vi "GEA2 Log Filter.vi"(0 "Filter Log":bool, 5 "Filter Data":bool, 7 "GEA2 Msg":T1 {"Command" format="%02x"; "Destination" format="%02x"; "Source" format="%02x"}, 9 "Cmd to Filter":string, 11 "error in (no error)":errorcluster) -> (15 "error out":errorcluster)   [LabVIEW 2021]
uses:
  Common/LabVIEW GEA2 Toolkit/GEA3/type defs/Data In.ctl
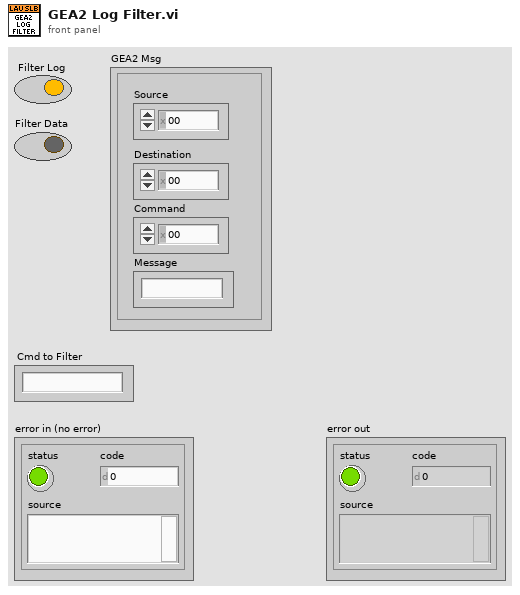
[diagram p1: front panel]
types:
  T1 = typedef "Data In.ctl" = cluster{"Source":u8, "Destination":u8, "Command":u8, "Message":string}
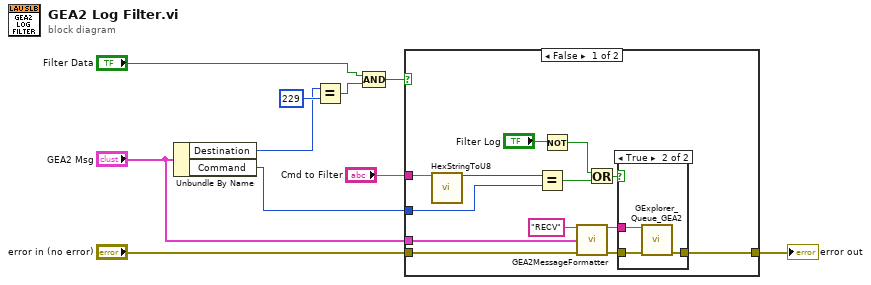
[diagram p0: block diagram]
diagram:
  n1 = Unbundle By Name("GEA2 Msg") -> ("Destination"=w3:u8, "Command"=w2:u8)
  n2 = Equal?(x=w3, y=u8 229) -> (x = y?=w8:bool)
  n3 = Compound Arithmetic op=AND("Filter Data", w8) -> (w9:bool)
  n4 = case shown="False" w9 {
    tunnel: "error in (no error)" -> [w14 w28]
    tunnel: [w23 w28] -> w6
    tunnel: w2 -> [w21 _]
    tunnel: "Cmd to Filter" -> [w17 _]
    tunnel: "GEA2 Msg" -> [w13 _]
    frame False {
      n5 = call "HexStringToU8.vi"("Input String"=w17) -> ("Number Out"=w22:u8)  [unwired: 14 in]
      n6 = Equal?(x=w22, y=w21) -> (x = y?=w20:bool)
      n7 = Not(x="Filter Log") -> (.not. x?=w18:bool)
      n8 = call "GEA2MessageFormatter.vi"("Prefix(Send/Recv)"="RECV", "GEA2 Data In"=w13, "Error In"=w14) -> ("Output String"=w15:string, "Error Out"=w16:errorcluster)  [unwired: 11 in]
      n9 = Or(x=w18, y=w20) -> (x .or. y?=w19:bool)
      n10 = case shown="True" w19 {
        tunnel: w16 -> [w24 w27]
        tunnel: [w24 w26] -> w23
        tunnel: w15 -> [_ w25]
        frame False {
        }
        frame True {
          n11 = call "GExplorer_Queue_GEA2.vi"("Output String"=w25, "error in (no error)"=w27) -> ("error out"=w26:errorcluster)  [unwired: 13 in]
        }
      }
    }
    frame True {
    }
  }
  "error out" <- w6
